vi "Get Available IP List - Multi FPGA.vi"(8 "error in (no error)":errorcluster, 10 "rio names":string[](array[string]), 11 "Item Ref in":T1 format="%.0x") -> (0 "error out":errorcluster, 2 "ips available":string[](array[string]), 3 "Item Ref out":T1 format="%.0x")   [LabVIEW 2015, in "Engine Simulation Toolkit System Explorer.lvlib"]
uses:
  Engine Simulation Toolkit System Explorer.lvlib
  <vilib>/NI Veristand/Custom Device API/Custom Device Item Ref.ctl
  <vilib>/NI Veristand/Custom Device Tools/Custom Device Utility Library/Search Direction.ctl
  Shared/Constants and GUIDs.vi
  <vilib>/NI Veristand/Custom Device Tools/Custom Device Utility Library/NI VeriStand - Search for Item by GUID.vi
  <vilib>/NI Veristand/Custom Device API/Get Item Property (String Array).vi
  <userlib>/_OpenG.lib/array/array.llb/Remove Duplicates from 1D Array (String)__ogtk.vi
  <vilib>/NI Veristand/Custom Device Tools/Custom Device Utility Library/Custom Device Utility Library.lvlib
  Shared/Engine Simulation Toolkit Shared.lvlib
  <vilib>/NI Veristand/Custom Device API/Custom Device API.lvlib
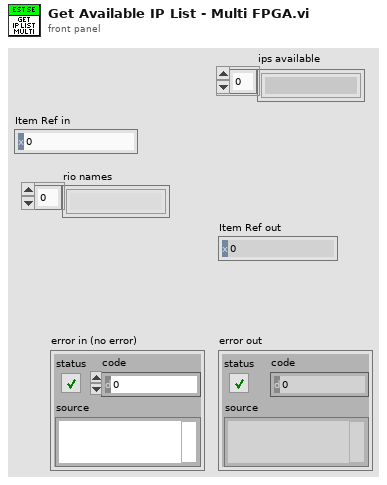
[diagram p1: front panel]
types:
  T1 = typedef "Custom Device API.lvlib/Custom Device Item Ref.ctl" = u64
  T2 = typedef "Custom Device Utility Library.lvlib/Search Direction.ctl" = enum16{"Down", "Up"}
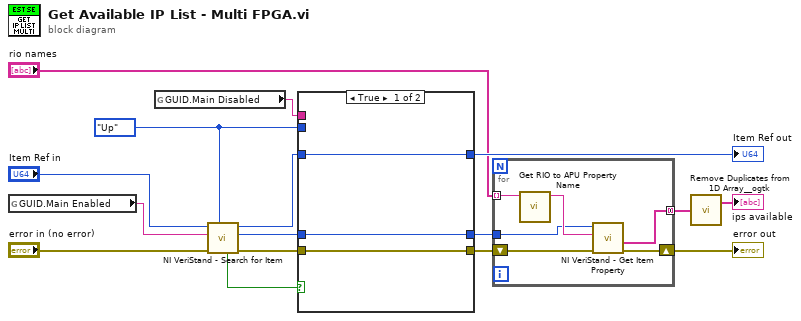
[diagram p0: block diagram]
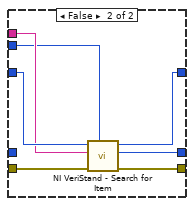
[diagram p2: hidden frame]
diagram:
  w8 = Search_Direction."Up" ("Direction (Down)")
  n1 = global read "Constants and GUIDs.vi" "GUID.Main Enabled"() -> (w14:string)
  n2 = global read "Constants and GUIDs.vi" "GUID.Main Disabled"() -> (w9:string)
  n3 = call-poly <vilib>:"NI VeriStand - Search for Item.vi"("Direction (Down)"=w8, "error in"="error in (no error)", "Item GUID"=w14, "Section Ref in"="Item Ref in") -> ("error out"=w12:errorcluster, "Item Ref"=w10:T1, "Section Ref out"=w11:T1, "Found"=w13:bool)  [unwired: 4 in]
  n4 = case shown="True" w13 {
    tunnel: w12 -> [w19 w26]
    tunnel: w11 -> [w17 w25]
    tunnel: w10 -> [w18 _]
    tunnel: w9 -> [_ w24]
    tunnel: w8 -> [_ w23]
    tunnel: [w18 w22] -> w5
    tunnel: [w17 w21] -> w7
    tunnel: [w19 w20] -> w4
    frame True {
    }
    frame False {
      n5 = call-poly <vilib>:"NI VeriStand - Search for Item.vi"("Direction (Down)"=w23, "error in"=w26, "Item GUID"=w24, "Section Ref in"=w25) -> ("error out"=w20:errorcluster, "Item Ref"=w22:T1, "Section Ref out"=w21:T1)  [unwired: 4 in, 1 out]
    }
  }
  "Item Ref out" <- w7
  n6 = for {
    tunnel: "rio names" -> [w32] mode=indexing
    tunnel: w5 -> [w30]
    shift-right: [w28] -> w3
    shift-left: w4 -> [w29]
    tunnel: [w27] -> w2 mode=concatenating
    n7 = call "Get RIO to APU Property Name.vi"("rio name"=w32) -> ("property name"=w31:string)  [unwired: 10 in]
    n8 = call-poly <vilib>:"NI VeriStand - Get Item Property.vi"("error in (no error)"=w29, "Property Name"=w31, "Item Ref in"=w30) -> ("error out"=w28:errorcluster, "Value"=w27:string[])  [unwired: 5 in, 2 out]
  }
  "error out" <- w3
  n9 = call-poly <userlib>:"Remove Duplicates from 1D Array__ogtk.vi"("Input Array"=w2) -> ("Output Array"=→"ips available":string[])  [unwired: 1 out]
